vi "Get Number of Color Transform Matrices.vi"(8 "error in (no error)":errorcluster, 11 "ColorProcessor reference in":refnum<k24>) -> (0 "error out":errorcluster, 2 "NumberOfColorTransformMatrices":i32, 3 "ColorProcessor reference out":refnum<k24>)   [LabVIEW 2015]
uses:
  C:/code/Host/Installer/Scientific Camera Interfaces/LabVIEW/64_bit/Library_X64/Thorlabs.TSI.ColorInterfaces.dll
  code/Host/Installer/Scientific Camera Interfaces/LabVIEW/64_bit/Library_X64/Thorlabs.TSI.ColorInterfaces.dll
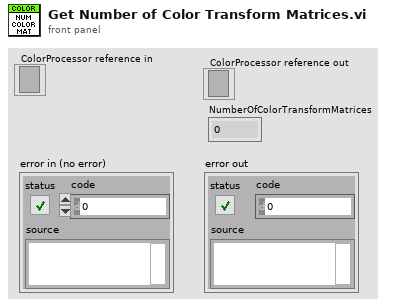
[diagram p1: front panel]
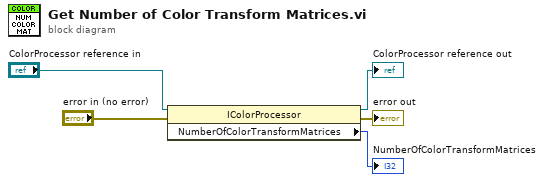
[diagram p0: block diagram]
diagram:
  n1 = property class="IColorProcessor"(reference="ColorProcessor reference in", error in="error in (no error)") -> (reference out=→"ColorProcessor reference out":refnum<k24>, error out=→"error out":errorcluster, "NumberOfColorTransformMatrices"=→"NumberOfColorTransformMatrices":i32)
